vi "MaxZ.vi"(8 "dwell_time_ms":dbl=100.0, 9 "q_steps":u32=100, 10 "z_end_um":dbl=100.0, 11 "z_start_um":dbl) -> (1 "mse":dbl, 2 "focus_data":T1(graph), 3 "z_focus_um":dbl)   [LabVIEW 2018]
uses:
  <vilib>/Analysis/1siggen.llb/Ramp Pattern by Samples.vi
  <vilib>/Analysis/NI_AALBase.lvlib
  <vilib>/Analysis/NI_AALPro.lvlib
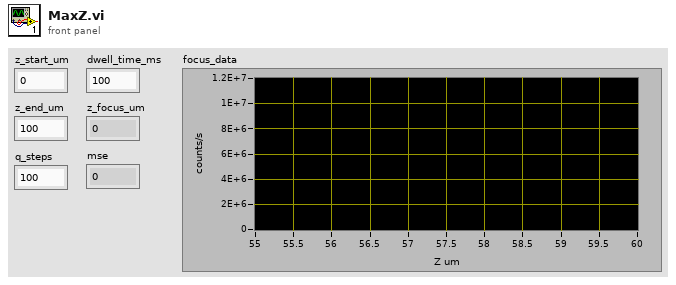
[diagram p1: front panel]
types:
  T1 = cluster{"Ramp Pattern":dbl[], "Best Gaussian Fit":dbl[]}[]
  T2 = cluster{"Ramp Pattern":dbl[], "Best Gaussian Fit":dbl[]}
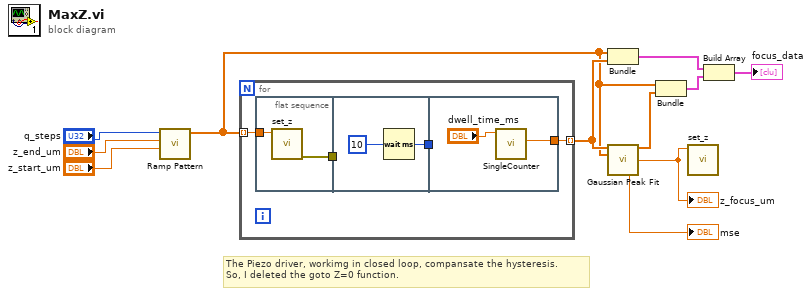
[diagram p0: block diagram]
diagram:
  # "The Piezo driver, workimg in closed loop, compansate the hysteresis.\nSo, I deleted the goto Z=0 function."
  n1 = call-poly <vilib>:"Ramp Pattern.vi"("start"="z_start_um", "end"="z_end_um", "samples"="q_steps") -> ("Ramp Pattern"=w5:dbl[])  [unwired: 7 in, 1 out]
  n2 = for {
    tunnel: w5 -> [w15] mode=indexing
    tunnel: [w14] -> w7 mode=indexing
    n3 = flat-sequence {
      tunnel: w15 -> [w17]
      tunnel: [w16] -> w13
      tunnel: w13 -> [_]
      tunnel: [w18] -> w12
      tunnel: [w20] -> w14
      tunnel: w12 -> [_]
      frame #0 {
        n4 = call "set_z.vi"("z_value_um"=w17) -> ("error out"=w16:errorcluster)  [unwired: 10 in]
      }
      frame #1 {
        n5 = Wait (ms)(milliseconds to wait=u32 10) -> (millisecond timer value=w18:u32)
      }
      frame #2 {
        n6 = call "SingleCounter.vi"("Dwell_time_ms"="dwell_time_ms") -> ("counts/s"=w20:dbl)  [unwired: 8 in, 2 out]
      }
    }
  }
  n7 = Bundle("Ramp Pattern"=w5, w7) -> (w4:cluster{"Ramp Pattern":dbl[], dbl[]})  [unwired: 1 in]
  n8 = call <vilib>:"Gaussian Peak Fit.vi"("Y"=w7, "X"=w5) -> ("Best Gaussian Fit"=w6:dbl[], "center"=w8:dbl, "residue"=→"mse":dbl)  [unwired: 7 in, 4 out]
  "z_focus_um" <- w8
  n9 = Bundle("Ramp Pattern"=w5, "Best Gaussian Fit"=w6) -> (w3:T2)  [unwired: 1 in]
  n10 = call "set_z.vi"("z_value_um"=w8) -> ()  [unwired: 10 in, 1 out]
  n11 = Build Array(w4, w3) -> (→"focus_data":T1)
